vi "Read common.vi"(8 "error in (no error)":errorcluster, 11 "tcv in":refnum<class "tcv.lvclass">) -> (0 "error out":errorcluster, 2 "common":T1={"tcv"=0, "Path"=path "", "resourcePath"="C:\\Program Files\\ADS\\Resources\\TCV_Lib.dll", "device"=enum."CPU"} {"tcv" format="%.0g"}, 3 "tcv out":refnum<class "tcv.lvclass">)   [LabVIEW 2025, in "tcv.lvlib" / "tcv.lvclass"]
uses:
  tcv.lvclass
  def/common.ctl
  def/devices.ctl
  tcv.lvclass/tcv.ctl
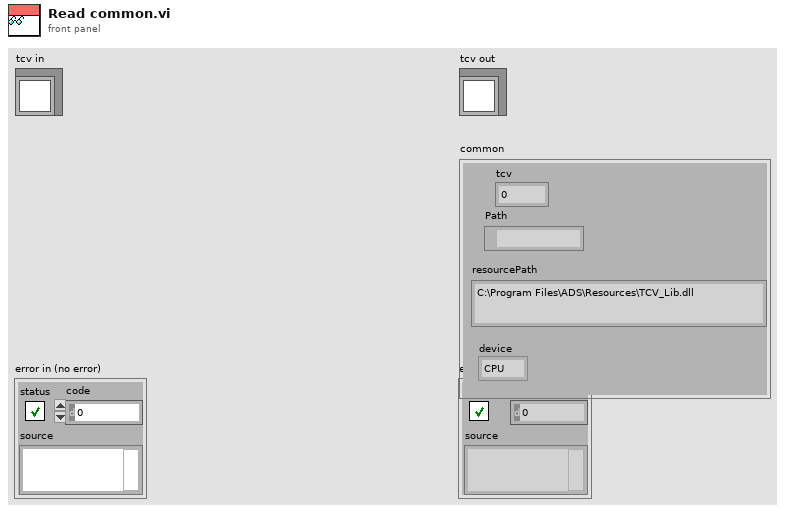
[diagram p1: front panel]
types:
  T1 = typedef "tcv.lvlib/tcv.lvclass/common.ctl" = cluster{"tcv":u64, "Path":path, "resourcePath":string, "device":T2}
  T2 = typedef "tcv.lvlib/tcv.lvclass/devices.ctl" = enum16{"CPU", "GPU0"}
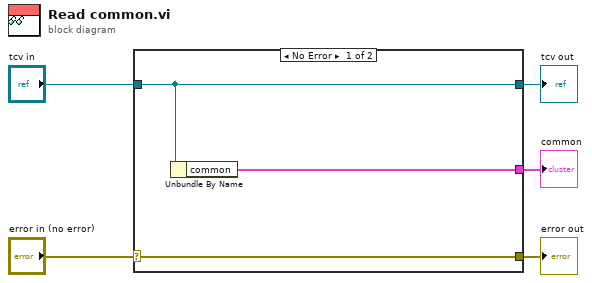
[diagram p0: block diagram]
diagram:
  n1 = case shown="No Error" "error in (no error)" {
    selector: "error in (no error)" -> [w8 w9]
    tunnel: [w8 w9] -> w4
    tunnel: [w7 w10] -> w2
    tunnel: "tcv in" -> [w7 w10]
    tunnel: [w6 _] -> w1
    frame No Error {
      n2 = Unbundle By Name(w7) -> ("common"=w6:T1)
    }
    frame Error {
    }
  }
  "error out" <- w4
  "tcv out" <- w2
  "common" <- w1
